vi "Test Inicializar Osciloscopio.vi"() -> ()   [LabVIEW 2020]
uses:
  <vilib>/addons/_JKI Toolkits/Caraya/classes/Assert/Assert True.vi
  <vilib>/addons/_JKI Toolkits/Caraya/classes/Test/Test.lvclass
  <vilib>/addons/_JKI Toolkits/Caraya/classes/Assert/Assert.lvclass
panel:
  out "Pass":bool
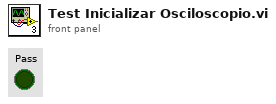
[diagram p1: front panel]
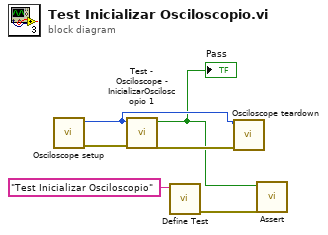
[diagram p0: block diagram]
diagram:
  n1 = call "Osciloscope setup.vi"() -> ("error out"=w5:errorcluster, "Module ID"=w4:i32)  [unwired: 10 in]
  n2 = call "Test - Osciloscope - InicializarOsciloscopio 1.vi"("error in (no error)"=w5, "Module ID"=w4) -> ("error out"=w6:errorcluster, "Pass"=w2:bool)  [unwired: 8 in]
  "Pass" <- w2
  n3 = call <vilib>:"Define Test.vi"("Label (VI Title)"="Test Inicializar Osciloscopio") -> ("error out"=w3:errorcluster)  [unwired: 10 in]
  n4 = call "Osciloscope teardown.vi"("error in"=w6, "Module ID"=w4) -> ()  [unwired: 9 in, 1 out]
  n5 = call-poly <vilib>:"Assert.vi"("error in (no error)"=w3, "True?"=w2) -> ()  [unwired: 9 in, 1 out]
